vi "PH_Beckhoff_PP_PU.handle Ignitrons.vi"(0 "i ref in":refnum<vi>, 4 "Values":T2, 5 "error in":errorcluster, 7 "Values changed at":T1) -> (14 "i ref out":refnum<vi>, 19 "error out":errorcluster)   [LabVIEW 2014, in "PH_Beckhoff_PP_PU.lvlib"]
doc: "This VI handles the incoming information about Ignitron inputs: The status is calculated and, if it changed, set to own attributes and published via DIM. All information is indicated at the GUI."
uses:
  PH_Beckhoff_PP_PU.lvlib
  PH_Beckhoff/PH_Beckhoff.Values.ctl
  PH_Beckhoff/PH_Beckhoff.Sonderklemmen Inputs.ctl
  PH_Beckhoff/PH_Beckhoff.Analog Inputs.ctl
  PH_Beckhoff/PH_Beckhoff.Scaling Type.ctl
  PH_Beckhoff/PH_Beckhoff.Analog Outputs.ctl
  PH_Beckhoff/PH_Beckhoff.Digital Inputs.ctl
  PH_Beckhoff/PH_Beckhoff.Digital Outputs.ctl
  PH_Basics/PH_StatusHandler/PH_StatusHandler.lvlib
  PH_Basics/PH_Common/PH_Common.lvlib
  PH_Beckhoff/PH_Beckhoff.lvlib
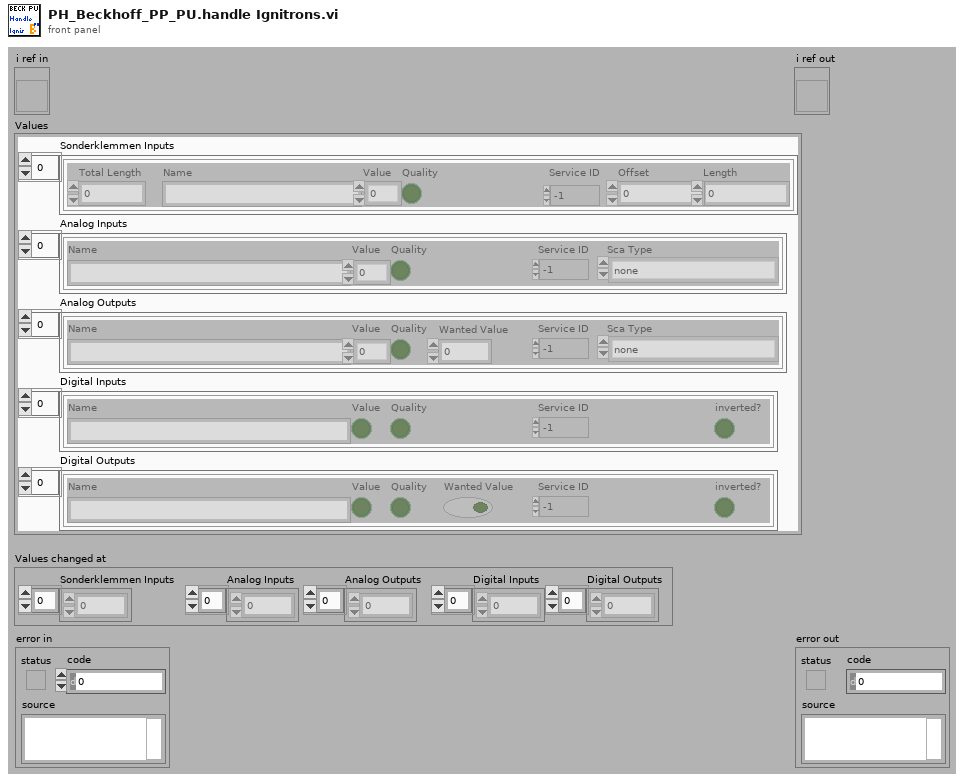
[diagram p1: front panel]
types:
  T1 = cluster{"Sonderklemmen Inputs":i32[], "Analog Inputs":i32[], "Analog Outputs":i32[], "Digital Inputs":i32[], "Digital Outputs":i32[]}
  T2 = typedef "PH_Beckhoff.lvlib/PH_Beckhoff.Values.ctl" = cluster{"Sonderklemmen Inputs":T3, "Analog Inputs":T4, "Analog Outputs":T6, "Digital Inputs":T7, "Digital Outputs":T8}
  T3 = typedef "PH_Beckhoff.lvlib/PH_Beckhoff.Sonderklemmen Inputs.ctl" = cluster{"Total Length":u32, "Name":string, "Value":u64, "Quality":bool, "Service ID":i32, "Offset":u32, "Length":u32}[]
  T4 = typedef "PH_Beckhoff.lvlib/PH_Beckhoff.Analog Inputs.ctl" = cluster{"Name":string, "Value":u32, "Quality":bool, "Service ID":i32, "Sca Type":T5}[]
  T5 = typedef "PH_Beckhoff.lvlib/PH_Beckhoff.Scaling Type.ctl" = enum16{"none", "0 ... 15 Bit -> 0 ... 5", "0 ... 15 Bit -> 0 ... 10", "0 ... 15 Bit -> 0 ... 25", "0 ... 15 Bit -> 4 ... 20", "0 ... 15 Bit -> 0 ... 1", "0 ... 15 Bit -> 0 ... 20000", "0 ... 15 Bit -> 0 ... 24000"}
  T6 = typedef "PH_Beckhoff.lvlib/PH_Beckhoff.Analog Outputs.ctl" = cluster{"Name":string, "Value":u32, "Quality":bool, "Wanted Value":u32, "Service ID":i32, "Sca Type":T5}[]
  T7 = typedef "PH_Beckhoff.lvlib/PH_Beckhoff.Digital Inputs.ctl" = cluster{"Name":string, "Value":bool, "Quality":bool, "Service ID":i32, "inverted?":bool}[]
  T8 = typedef "PH_Beckhoff.lvlib/PH_Beckhoff.Digital Outputs.ctl" = cluster{"Name":string, "Value":bool, "Quality":bool, "Wanted Value":bool, "Service ID":i32, "inverted?":bool}[]
  T9 = typedef "PH_Beckhoff_PP_PU.lvlib/PH_Beckhoff_PP_PU.PU Rack Type.ctl" = enum16{"no Info", "PA 19mm", "PA 45mm", "MA PU 1 and 2", "MA PU 3 and 4", "MA PU 5 and 6", "MA FR and PILC"}
  T10 = typedef "PH_Beckhoff_PP_PU.lvlib/PH_Beckhoff_PP_PU.i attribute.ctl" = cluster{"HV Meas":cluster{"Input GUI Ref":refnum<vi>, "Voltage Service ID":i32, "Voltage [V]":dbl, "Quality":bool, "# in Data":i32}[], "Trigger":cluster{"Status":cluster{"GUI Ref":refnum<vi>, "Status Service ID":i32, "Status":T11}, "last shot:":cluster{"GUI Ref":refnum<vi>, "Service ID":i32, "Time":string}, "DIs":cluster{"triggered":cluster{"GUI Ref":refnum<vi>, "# in Data":i32}, "fired":cluster{"GUI Ref":refnum<vi>, "# in Data":i32}}, "GUI Ref Indicator":refnum<vi>}[], "RR":cluster{"Status":cluster{"GUI Ref":refnum<vi>, "Status Service ID":i32, "Status":T11}, "DIs":cluster{"closed":cluster{"GUI Ref":refnum<vi>, "# in Data":i32}, "open":cluster{"GUI Ref":refnum<vi>, "# in Data":i32}}, "Close":cluster{"GUI Ref":refnum<vi>, "# in Data":i32}, "GUI Ref Indicator":refnum<vi>}[], "Igni":cluster{"Status":cluster{"GUI Ref":refnum<vi>, "Status Service ID":i32, "Status":T11}, "DIs":cluster{"heating on":cluster{"GUI Ref":refnum<vi>, "# in Data":i32}, "water on":cluster{"GUI Ref":refnum<vi>, "# in Data":i32}}, "Device on":cluster{"GUI Ref":refnum<vi>, "# in Data":i32}, "GUI Ref Indicator":refnum<vi>}[], "PSU":cluster{"Status":cluster{"GUI Ref":refnum<vi>, "Status Service ID":i32, "Status":T11}, "Limit Service ID":i32, "DIs":cluster{"inhibit":cluster{"GUI Ref":refnum<vi>, "# in Data":i32}, "end of charge":cluster{"GUI Ref":refnum<vi>, "# in Data":i32}, "HV on":cluster{"GUI Ref":refnum<vi>, "# in Data":i32}, "overtemp":cluster{"GUI Ref":refnum<vi>, "# in Data":i32}, "interlock":cluster{"GUI Ref":refnum<vi>, "# in Data":i32}, "load fault":cluster{"GUI Ref":refnum<vi>, "# in Data":i32}, "sum fault":cluster{"GUI Ref":refnum<vi>, "# in Data":i32}, "HV off":cluster{"GUI Ref":refnum<vi>, "# in Data":i32}, "DC ok":cluster{"GUI Ref":refnum<vi>, "# in Data":i32}}, "AIs":cluster{"voltage":cluster{"GUI Ref":refnum<vi>, "# in Data":i32}, "current":cluster{"GUI Ref":refnum<vi>, "# in Data":i32}}, "DAs":cluster{"inhibit":cluster{"GUI Ref":refnum<vi>, "# in Data":i32}, "interlock":cluster{"GUI Ref":refnum<vi>, "# in Data":i32}, "HV on":cluster{"GUI Ref":refnum<vi>, "# in Data":i32}, "Reset":cluster{"GUI Ref":refnum<vi>, "# in Data":i32}}, "AAs":cluster{"Voltage to set":cluster{"GUI Ref":refnum<vi>, "# in Data":i32}}, "GUI Ref Indicator":refnum<vi>}[], "reconfigured":cluster{"?":bool, "GUI Ref":refnum<vi>}, "PU Rack Type":T9, "HV Meas Info":T12, "PSU Info":T13}
  T11 = typedef "PH_StatusHandler.lvlib/PH_StatusHandler.Status.ctl" = i16
  T12 = typedef "PH_Beckhoff_PP_PU.lvlib/PH_Beckhoff_PP_PU.HV Meas Info.ctl" = cluster{"Period Time [s]":dbl, "Subtractor 1 [Hz]":dbl, "Devider 1 [Hz/kV]":dbl, "Subtractor 2 [Hz]":dbl, "Devider 2 [Hz/kV]":dbl}
  T13 = typedef "PH_Beckhoff_PP_PU.lvlib/PH_Beckhoff_PP_PU.PSU Info.ctl" = cluster{"Limits 1 [V]":cluster{"Lower":dbl, "Upper":dbl}, "Limits 2 [V]":cluster{"Lower":dbl, "Upper":dbl}}
  T14 = cluster{"Status":cluster{"GUI Ref":refnum<vi>, "Status Service ID":i32, "Status":T11}, "DIs":cluster{"heating on":cluster{"GUI Ref":refnum<vi>, "# in Data":i32}, "water on":cluster{"GUI Ref":refnum<vi>, "# in Data":i32}}, "Device on":cluster{"GUI Ref":refnum<vi>, "# in Data":i32}, "GUI Ref Indicator":refnum<vi>}[]
  T15 = cluster{"Status":cluster{"GUI Ref":refnum<vi>, "Status Service ID":i32, "Status":T11}, "DIs":cluster{"heating on":cluster{"GUI Ref":refnum<vi>, "# in Data":i32}, "water on":cluster{"GUI Ref":refnum<vi>, "# in Data":i32}}, "Device on":cluster{"GUI Ref":refnum<vi>, "# in Data":i32}, "GUI Ref Indicator":refnum<vi>}
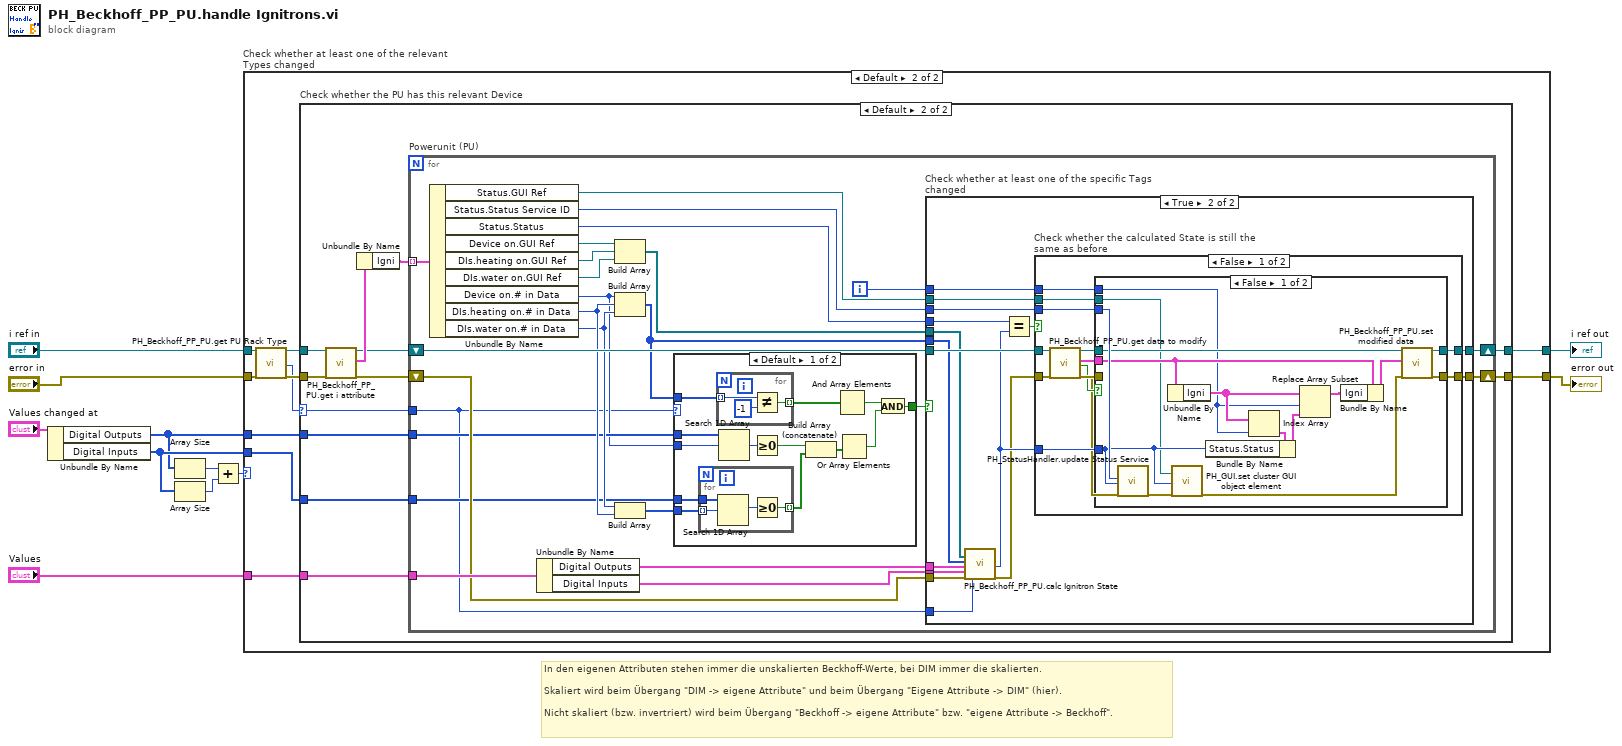
[diagram p0: block diagram]
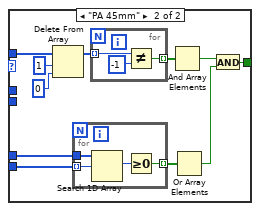
[diagram p4: hidden frame]
diagram:
  # "In den eigenen Attributen stehen immer die unskalierten Beckhoff-Werte, bei DIM immer die skalierten.\n\nSkaliert wird beim Übergang \"DIM -> eigene Attribute\" und beim Übergang \"Eigene Attribute -> DIM\" (hier).\n\nNicht skaliert (bzw. invertriert) wird beim Übergang \"Beckhoff -> eigene Attribute\" bzw. \"eigene Attribute -> Beckhoff\"."
  n1 = Unbundle By Name("Values changed at") -> ("Digital Outputs"=w1:i32[], "Digital Inputs"=w2:i32[])
  n2 = Array Size(array=w1) -> (size(s)=w5:i32)
  n3 = Array Size(array=w2) -> (size(s)=w4:i32)
  n4 = Add(x=w5, y=w4) -> (x+y=w3:i32)
  n5 = case "Check whether at least one of the relevant Types changed" shown="Default" w3 {
    tunnel: [w12 w21] -> w11
    tunnel: "i ref in" -> [w13 w18]
    tunnel: "error in" -> [w12 w16]
    tunnel: "Values" -> [_ w22]
    tunnel: [w13 w23] -> w7
    tunnel: w2 -> [_ w20]
    tunnel: w1 -> [_ w19]
    frame 0 {
    }
    frame Default {
      n6 = call "PH_Beckhoff_PP_PU.get PU Rack Type.vi"("VI in"=w18, "error in (no error)"=w16) -> ("VI out"=w17:refnum<vi>, "PU Rack Type"=w14:T9, "error out"=w15:errorcluster)  [unwired: 15 in]
      n7 = case "Check whether the PU has this relevant Device" shown="Default" w14 {
        selector: w14 -> [_ w26]
        tunnel: [w25 w37] -> w23
        tunnel: w22 -> [_ w36]
        tunnel: [w24 w33] -> w21
        tunnel: w20 -> [_ w32]
        tunnel: w19 -> [_ w31]
        tunnel: w17 -> [w25 w28]
        tunnel: w15 -> [w24 w27]
        frame "no Info", "PA 19mm" {
        }
        frame Default {
          n8 = call "PH_Beckhoff_PP_PU.get i attribute.vi"("i ref in"=w28, "error in (no error)"=w27) -> ("i ref out"=w30:refnum<vi>, "i attribute"=w35:T10, "error out"=w29:errorcluster)  [unwired: 15 in]
          n9 = Unbundle By Name(w35) -> ("Igni"=w34:T14)
          n10 = for "Powerunit (PU)" {
            shift-right: [w56] -> w33
            shift-left: w29 -> [w47]
            tunnel: w34 -> [w62] mode=indexing
            shift-right: [w57] -> w37
            shift-left: w30 -> [w59]
            tunnel: w36 -> [w54]
            tunnel: w32 -> [w42]
            tunnel: w31 -> [w41]
            tunnel: w26 -> [w38]
            i -> [w58]
            n11 = Unbundle By Name(w62) -> ("Status.GUI Ref"=w52:refnum<vi>, "Status.Status Service ID"=w61:i32, "Status.Status"=w60:T11, "Device on.GUI Ref"=w51:refnum<vi>, "DIs.heating on.GUI Ref"=w50:refnum<vi>, "DIs.water on.GUI Ref"=w49:refnum<vi>, "Device on.# in Data"=w40:i32, "DIs.heating on.# in Data"=w44:i32, "DIs.water on.# in Data"=w43:i32)
            n12 = Unbundle By Name(w54) -> ("Digital Outputs"=w53:T8, "Digital Inputs"=w55:T7)
            n13 = Build Array(w51, w50, w49) -> (w48:refnum<vi>[])
            n14 = Build Array(w40, w44, w43) -> (w46:i32[])
            n15 = Build Array(w43, w44) -> (w45:i32[])
            n16 = case shown="Default" w38 {
              tunnel: w46 -> [w72 w90]
              tunnel: w45 -> [w71 w89]
              tunnel: w42 -> [w70 w88]
              tunnel: w41 -> [w69 _]
              tunnel: w40 -> [w68 _]
              tunnel: [w64 w87] -> w39
              frame Default {
                n17 = for {
                  tunnel: w70 -> [w79]
                  tunnel: [w78] -> w66 mode=indexing
                  tunnel: w71 -> [w77] mode=indexing
                  n18 = Search 1D Array(1D array=w79, element=w77) -> (index of element=w76:i32)  [unwired: 1 in]
                  n19 = Greater Or Equal To 0?(x=w76) -> (x >= 0?=w78:bool)
                }
                n20 = for {
                  tunnel: w72 -> [w81] mode=indexing
                  tunnel: [w82] -> w75 mode=indexing
                  n21 = Not Equal?(x=w81, y=-1) -> (x != y?=w82:bool)
                }
                n22 = Search 1D Array(1D array=w69, element=w68) -> (index of element=w63:i32)  [unwired: 1 in]
                n23 = Greater Or Equal To 0?(x=w63) -> (x >= 0?=w67:bool)
                n24 = Build Array (concatenate)(w67, w66) -> (w65:bool[])
                n25 = And Array Elements(Boolean array=w75) -> (logical AND=w74:bool)
                n26 = Or Array Elements(Boolean array=w65) -> (logical OR=w73:bool)
                n27 = And(x=w74, y=w73) -> (x .and. y?=w64:bool)
              }
              frame "PA 45mm" {
                n28 = Delete From Array(array=w90, length=1, index=0) -> (array with subset deleted=w85:i32[])  [unwired: 1 out]
                n29 = for {
                  tunnel: w88 -> [w97]
                  tunnel: [w96] -> w86 mode=indexing
                  tunnel: w89 -> [w95] mode=indexing
                  n30 = Search 1D Array(1D array=w97, element=w95) -> (index of element=w94:i32)  [unwired: 1 in]
                  n31 = Greater Or Equal To 0?(x=w94) -> (x >= 0?=w96:bool)
                }
                n32 = for {
                  tunnel: w85 -> [w99] mode=indexing
                  tunnel: [w100] -> w93 mode=indexing
                  n33 = Not Equal?(x=w99, y=-1) -> (x != y?=w100:bool)
                }
                n34 = And Array Elements(Boolean array=w93) -> (logical AND=w92:bool)
                n35 = Or Array Elements(Boolean array=w86) -> (logical OR=w91:bool)
                n36 = And(x=w92, y=w91) -> (x .and. y?=w87:bool)
              }
            }
            n37 = case "Check whether at least one of the specific Tags changed" shown="True" w39 {
              tunnel: w61 -> [_ w118]
              tunnel: w60 -> [_ w117]
              tunnel: w59 -> [w102 w116]
              tunnel: w58 -> [_ w115]
              tunnel: [w102 w114] -> w57
              tunnel: [w101 w113] -> w56
              tunnel: w55 -> [_ w112]
              tunnel: w53 -> [_ w111]
              tunnel: w52 -> [_ w109]
              tunnel: w48 -> [_ w108]
              tunnel: w47 -> [w101 w105]
              tunnel: w46 -> [_ w104]
              tunnel: w38 -> [_ w103]
              frame False {
              }
              frame True {
                n38 = call "PH_Beckhoff_PP_PU.calc Ignitron State.vi"("GUI Refs: Device on, heating on, water on"=w108, "#: Device on, heating on, water on"=w104, "Digital Outputs"=w111, "Digital Inputs"=w112, "error in"=w105, "PU Type"=w103) -> ("Ignitron Status"=w107:T11, "error out"=w106:errorcluster)  [unwired: 12 in]
                n39 = Equal?(x=w117, y=w107) -> (x = y?=w110:bool)
                n40 = case "Check whether the calculated State is still the same as before" shown="False" w110 {
                  tunnel: [w125 w149] -> w113
                  tunnel: w118 -> [w130 _]
                  tunnel: w106 -> [w129 w149]
                  tunnel: w107 -> [w128 _]
                  tunnel: w116 -> [w126 w150]
                  tunnel: [w123 w150] -> w114
                  tunnel: w115 -> [w121 _]
                  tunnel: w109 -> [w119 _]
                  frame False {
                    n41 = call "PH_Beckhoff_PP_PU.get data to modify.vi"("i ref in"=w126, "error in (no error)"=w129) -> ("i ref out"=w124:refnum<vi>, "i attribute"=w122:T10, "timed out"=w120:bool, "error out"=w127:errorcluster)  [unwired: 14 in]
                    n42 = case shown="False" w120 {
                      tunnel: w130 -> [w146 _]
                      tunnel: w128 -> [w132 _]
                      tunnel: w127 -> [w145 w147]
                      tunnel: [w144 w147] -> w125
                      tunnel: w124 -> [w143 w148]
                      tunnel: [w142 w148] -> w123
                      tunnel: w122 -> [w141 _]
                      tunnel: w121 -> [w137 _]
                      tunnel: w119 -> [w131 _]
                      frame False {
                        n43 = call "PH_StatusHandler.update Status Service.vi"("Service ID"=w146, "Status"=w132, "error in (no error)"=w145) -> ("error out"=w134:errorcluster)  [unwired: 16 in]
                        n44 = Unbundle By Name(w141) -> ("Igni"=w138:T14)
                        n45 = call "PH_GUI.set cluster GUI object element.vi"("Ctl Refnum"=w131, "Value"=w132, "error in"=w134) -> ("error out"=w133:errorcluster)  [unwired: 16 in]
                        n46 = Index Array(array=w138, index=w137) -> (element=w136:T15)
                        n47 = Bundle By Name(cluster=w136, "Status.Status"=w132) -> (w135:T15)
                        n48 = Replace Array Subset(array=w138, new element=w135, index=w137) -> (w139:T14)
                        n49 = Bundle By Name(cluster=w141, "Igni"=w139) -> (w140:T10)
                        n50 = call "PH_Beckhoff_PP_PU.set modified data.vi"("i ref in"=w143, "i attribute"=w140, "error in (no error)"=w133) -> ("i ref out"=w142:refnum<vi>, "error out"=w144:errorcluster)  [unwired: 15 in]
                      }
                      frame True {
                      }
                    }
                  }
                  frame True {
                  }
                }
              }
            }
          }
        }
      }
    }
  }
  "error out" <- w11
  "i ref out" <- w7
